vi "AlignCameraFrame (SubVI).vi"(8 "error in (no error)":errorcluster, 10 "Image Src":T1, 11 "Refnum in":T2) -> (0 "error out":errorcluster, 2 "Image Dst Out":T1, 3 "Refnum out":T2)   [LabVIEW 2016]
uses:
  <vilib>/userdefined/High Color/IMAQdx.ctl
  <vilib>/vision/Image Controls.llb/IMAQ Image.ctl
  <resource>/objmgr/imaqdx.rc
  <vilib>/vision/NI_Vision_Development_Module.lvlib
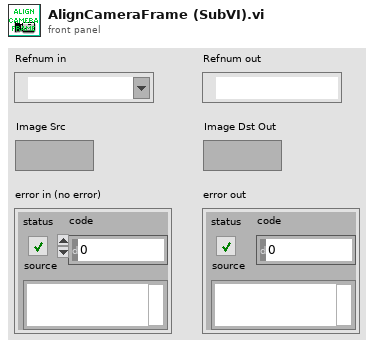
[diagram p1: front panel]
types:
  T1 = typedef "IMAQ Image.ctl" = refnum<image>
  T2 = typedef "IMAQdx.ctl" = refnum<k21>
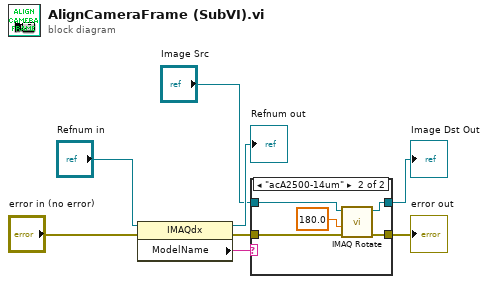
[diagram p0: block diagram]
diagram:
  n1 = property class="IMAQdx"(reference="Refnum in", error in="error in (no error)") -> (reference out=→"Refnum out":T2, error out=w8:errorcluster, "ModelName"=w1:string)
  n2 = case shown="\"acA2500-14um\"" w1 {
    tunnel: w8 -> [w9 w14]
    tunnel: [w9 w13] -> w2
    tunnel: [w10 w12] -> w3
    tunnel: "Image Src" -> [w10 w11]
    frame "acA3800-14um", Default {
    }
    frame "acA2500-14um" {
      n3 = call "IMAQ Rotate"("error in (no error)"=w14, "Angle (degrees)"=sgl 180.0, "Image Src"=w11) -> ("error out"=w13:errorcluster, "Image Dst Out"=w12:T1)  [unwired: 7 in]
    }
  }
  "Image Dst Out" <- w3
  "error out" <- w2
